vi "LH_IndexFirstContentSearch.vi"(2 "TargetContent":i32, 3 "InputList":refnum<class "ListHead.lvclass">) -> (0 "ResIndex":i32, 1 "Output":refnum<class "ListHead.lvclass">)   [LabVIEW 2014, in "ListHead.lvclass"]
uses:
  ListHead.lvclass
  ListHead.lvclass/ListHead.ctl
  ListNode.lvclass
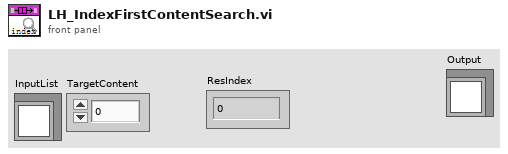
[diagram p1: front panel]
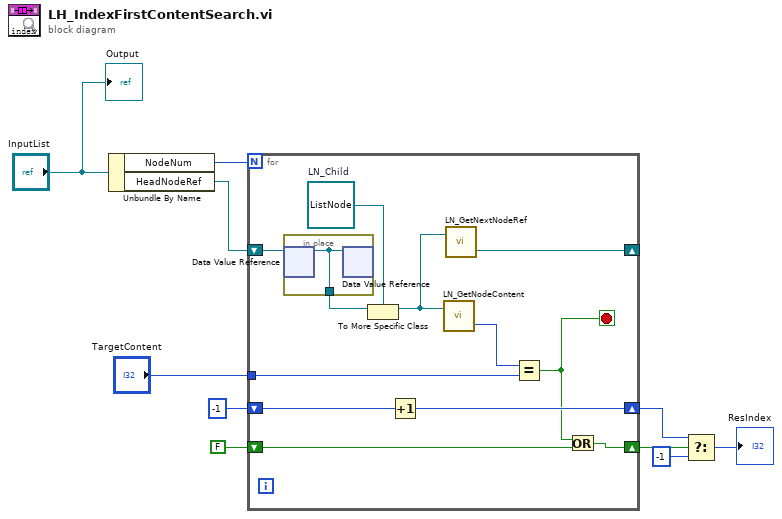
[diagram p0: block diagram]
diagram:
  n1 = Unbundle By Name("InputList") -> ("NodeNum"=w9:u32, "HeadNodeRef"=w8:refnum<data-value>)
  n2 = for {
    N: w9 -> [_]
    shift-right: [w16] -> _
    shift-left: w8 -> [w22]
    tunnel: "TargetContent" -> [w19]
    shift-right: [w14] -> w3
    shift-left: -1 ("f") -> [w15]
    shift-right: [w11] -> w4
    shift-left: FALSE -> [w13]
    stop <- w12 stop-if-true
    w20 = refnum<class "ListNode.lvclass"> refnum  # LN_Child
    n3 = in-place {
      in-place-border: [w23] -> w21
      n4 = in-place-dvr #1(w22) -> (w23:refnum<class "ListNodeVirtual.lvclass">)  [unwired: 1 out]
      n5 = in-place-dvr #1(w23) -> ()  [unwired: 2 out]
    }
    n6 = To More Specific Class(target class=w20, reference=w21) -> (specific class reference=w17:refnum<class "ListNode.lvclass">)  [unwired: 1 in, 1 out]
    n7 = Increment(x=w15) -> (x+1=w14:i32)
    n8 = call "LN_GetNodeContent.vi"("InputNode"=w17) -> ("Content"=w18:i32)  [unwired: 1 in, 1 out]
    n9 = call "LN_GetNextNodeRef.vi"("InputListNode"=w17) -> ("OutputNextNodeRef"=w16:refnum<data-value>)  [unwired: 1 in, 1 out]
    n10 = Equal?(x=w18, y=w19) -> (x = y?=w12:bool)
    n11 = Or(x=w12, y=w13) -> (x .or. y?=w11:bool)
  }
  n12 = Select(t=w3, s=w4, f=-1) -> (s? t:f=→"ResIndex":i32)
  "Output" <- "InputList"
